vi "Create.vi"(8 "error in (no error)":errorcluster, 9 "Player2":refnum<class "Player.lvclass">, 10 "Player1":refnum<class "Player.lvclass">, 11 "Board":refnum<class "Board.lvclass">) -> (0 "error out":errorcluster, 3 "Game out":refnum<class "Game.lvclass">)   [LabVIEW 2015, in "TronviewGame.lvlib" / "Game.lvclass"]
uses:
  Game.lvclass
  Player/Player.lvclass
  Board/Board.lvclass
  Game.lvclass/Game.ctl
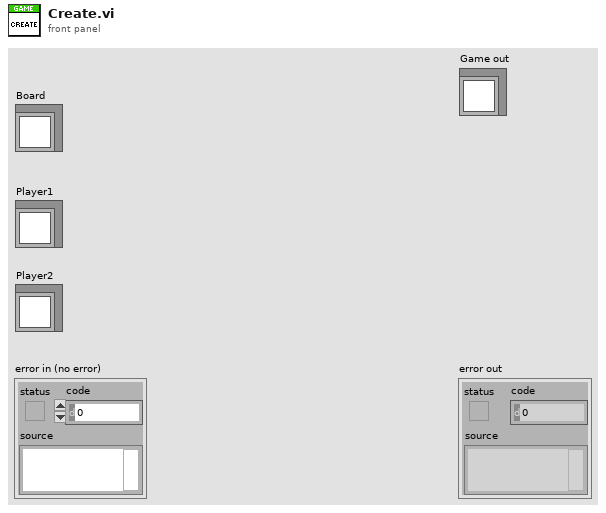
[diagram p1: front panel]
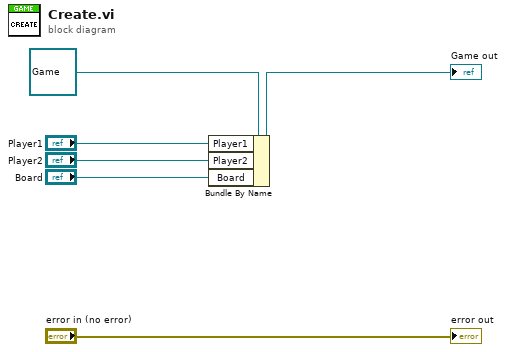
[diagram p0: block diagram]
diagram:
  n1 = Bundle By Name(cluster=refnum<class "Game.lvclass"> refnum ("Game in"), "Player1"="Player1", "Player2"="Player2", "Board"="Board") -> (→"Game out":refnum<class "Game.lvclass">)
  "error out" <- "error in (no error)"
